vi "pre-allocated_with_type.vi"(8 "error in (no error)":errorcluster, 11 "Test Data in":T1) -> (0 "error out":errorcluster, 3 "Test Data out":T1)   [LabVIEW 2024, in "IPE Optimization Tester.lvlib"]
uses:
  IPE Optimization Tester.lvlib
  test_data--cluster.ctl
  packetized_data--cluster.ctl
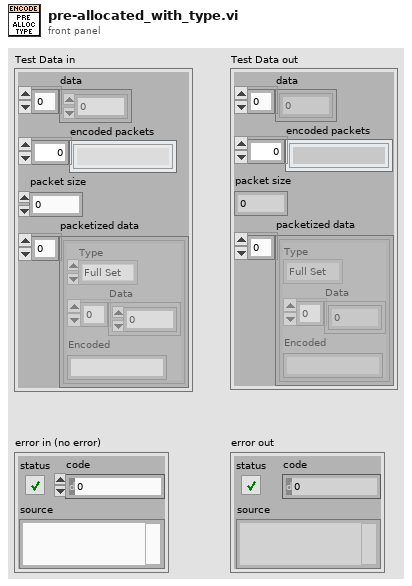
[diagram p1: front panel]
types:
  T1 = typedef "IPE Optimization Tester.lvlib/test_data--cluster.ctl" = cluster{"data":dbl[], "encoded packets":string[], "packet size":i32, "packetized data":T2[]}
  T2 = typedef "IPE Optimization Tester.lvlib/packetized_data--cluster.ctl" = cluster{"Type":enum16{"Full Set", "Last Set"}, "Data":dbl[], "Encoded":string}
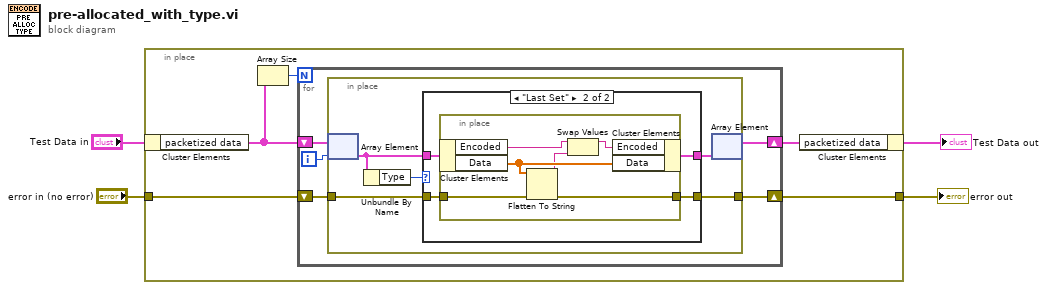
[diagram p0: block diagram]
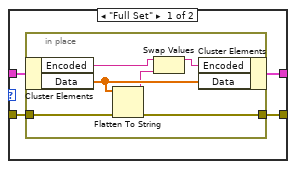
[diagram p2: hidden frame]
diagram:
  n1 = in-place {
    in-place-border: "error in (no error)" -> [w6]
    in-place-border: [w5] -> w2
    n2 = in-place-cluster #1("Test Data in") -> ("packetized data"=w8:T2[])
    n3 = Array Size(array=w8) -> (size(s)=w9:i32)
    n4 = for {
      N: w9 -> [_]
      shift-right: [w13] -> w7
      shift-left: w8 -> [w14]
      shift-right: [w12] -> w5
      shift-left: w6 -> [w11]
      i -> [w10]
      n5 = in-place {
        in-place-border: [w19] -> w12
        in-place-border: w11 -> [w18]
        n6 = in-place-array #2(w14, w10) -> (w16:T2)
        n7 = Unbundle By Name(w16) -> ("Type"=w15:enum16{"Full Set", "Last Set"})
        n8 = case shown="\"Last Set\"" w15 {
          tunnel: w16 -> [w23 w33]
          tunnel: [w22 w32] -> w19
          tunnel: w18 -> [w21 w31]
          tunnel: [w20 w30] -> w17
          frame "Full Set" {
            n9 = in-place {
              in-place-border: [w28] -> w22
              in-place-border: w21 -> [w27]
              n10 = in-place-cluster #3(w23) -> ("Encoded"=w25:string, "Data"=w29:dbl[])
              n11 = Flatten To String(anything=w29, error in (no error)=w27) -> (data string=w26:string, error out=w28:errorcluster)  [unwired: 2 in, 1 out]
              n12 = Swap Values(12:w25, 14:w26) -> (1:w24:string)  [unwired: 1 in, 1 out]
              n13 = in-place-cluster #3("Encoded"=w24, "Data"=w29) -> (w20:T2)
            }
          }
          frame "Last Set" {
            n14 = in-place {
              in-place-border: [w38] -> w32
              in-place-border: w31 -> [w37]
              n15 = in-place-cluster #4(w33) -> ("Encoded"=w35:string, "Data"=w39:dbl[])
              n16 = Flatten To String(anything=w39, error in (no error)=w37) -> (data string=w36:string, error out=w38:errorcluster)  [unwired: 2 in, 1 out]
              n17 = Swap Values(12:w35, 14:w36) -> (1:w34:string)  [unwired: 1 in, 1 out]
              n18 = in-place-cluster #4("Encoded"=w34, "Data"=w39) -> (w30:T2)
            }
          }
        }
        n19 = in-place-array #2(w17) -> (w13:T2[])  [unwired: 1 out]
      }
    }
    n20 = in-place-cluster #1("packetized data"=w7) -> (→"Test Data out":T1)
  }
  "error out" <- w2
